vi "Video Intro.vi"() -> ()   [LabVIEW 2012]
uses:
  SubVIs/LVPresent_Globals.vi
panel:
  in  "Seek Forward Button":bool
  in  "Seek Back Button":bool
  in  "Media Stop Button":bool
  in  "Pause Button":bool
  in  "Play Button":bool
  in  "Movie Path":path=path "/Macintosh HD/Users/Jenny/Dropbox/JumboBooks/JumboBooks/Talk/Movies/Video 4b.mov"
  out "Movie":picture
  # "Video Intro to LabVIEW"
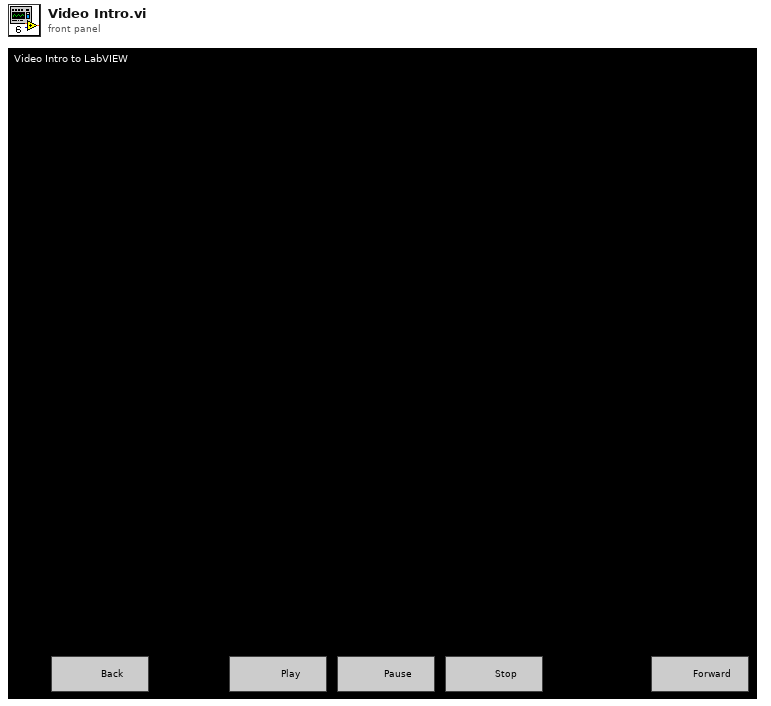
[diagram p1: front panel]
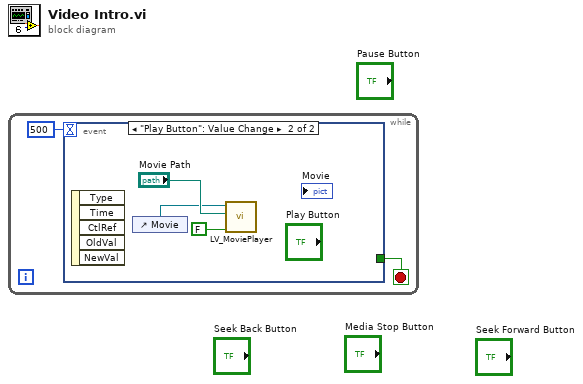
[diagram p0: block diagram]
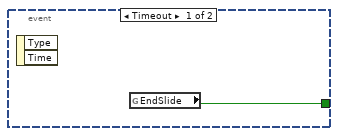
[diagram p2: hidden frame]
diagram:
  n1 = while {
    stop <- w2 stop-if-true
    n2 = event shown="[1] \"Play Button\": Value Change" {
      selector: _ -> [_ _]
      dyn-events: _ -> [_ _]
      timeout: 500 -> [_ _]
      tunnel: [w3 _] -> w2
      event Timeout {
        n3 = event-data() -> ()  [unwired: 1 in, 2 out]
        n4 = global read "LVPresent_Globals.vi" "EndSlide"() -> (w3:bool)
      }
      event "Play Button": Value Change {
        n5 = event-data() -> ()  [unwired: 1 in, 5 out]
        n6 = control-ref of="Movie"() -> (w4:refnum<vi>)
        n7 = call "LV_MoviePlayer.vi"("Play at maximum speed"=FALSE, "Movie Path"="Movie Path", "reference"=w4) -> ()  [unwired: 2 in, 1 out]
      }
    }
  }
